vi "OpenProcess.vi"(2 "process name":string, 4 "error in (no error)":errorcluster, 5 "bInheritHandle (0)":i32, 6 "dwDesiredAccesses (0)":i32, 7 "dwProcessId (0)":i32) -> (0 "error out":errorcluster, 3 "hProcess":i32)   [LabVIEW 2011]
uses:
  KERNEL32.DLL
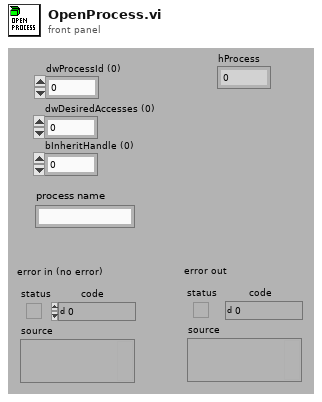
[diagram p1: front panel]
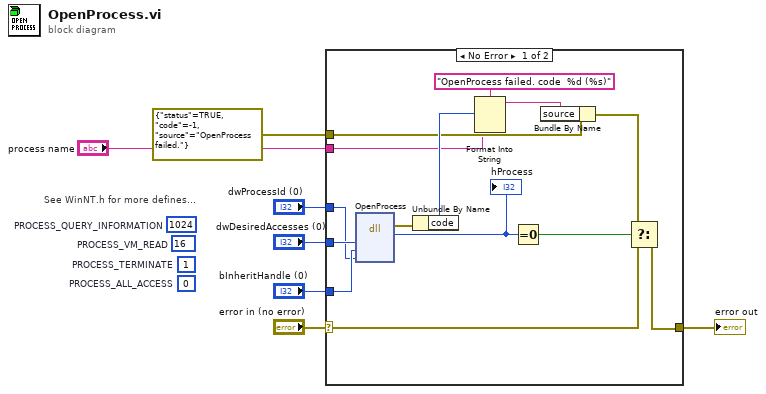
[diagram p0: block diagram]
diagram:
  (unwired) 1  # PROCESS_TERMINATE
  (unwired) 16  # PROCESS_VM_READ
  (unwired) 1024  # PROCESS_QUERY_INFORMATION
  (unwired) 0  # PROCESS_ALL_ACCESS
  # "See WinNT.h for more defines..."
  n1 = case shown="No Error" "error in (no error)" {
    selector: "error in (no error)" -> [w21 w22]
    tunnel: [w20 w22] -> w6
    tunnel: "bInheritHandle (0)" -> [w17 _]
    tunnel: "dwDesiredAccesses (0)" -> [w16 _]
    tunnel: "dwProcessId (0)" -> [w15 _]
    tunnel: errorcluster {"status"=TRUE, "code"=-1, "source"="OpenProcess failed."} ("error IO") -> [w10 _]
    tunnel: "process name" -> [w8 _]
    frame No Error {
      n2 = dll-call lib="KERNEL32.DLL" fn="OpenProcess"("dwDesiredAccessas"=w16, "bInheritHandle"=w17, "dwProcId"=w15) -> (error out=w12:errorcluster, "hProcess"=w19:i32)  [unwired: 6 in, 1 out]
      "hProcess" <- w19
      n3 = Unbundle By Name(w12) -> ("code"=w11:i32)
      n4 = Format Into String(format string="OpenProcess failed. code  %d (%s)" ("source"), w11, w8) -> (resulting string=w14:string)  [unwired: 2 in, 1 out]
      n5 = Equal To 0?(x=w19) -> (x = 0?=w18:bool)
      n6 = Bundle By Name(cluster=w10, "source"=w14) -> (w9:errorcluster)
      n7 = Select(t=w9, s=w18, f=w21) -> (s? t:f=w20:errorcluster)
    }
    frame Error {
    }
  }
  "error out" <- w6
